vi "Obsever Structure.vi"(8 "error in (no error)":errorcluster, 11 "Vessel in":refnum<class "Vessel.lvclass">) -> (0 "error out":errorcluster, 3 "Vessel out":refnum<class "Vessel.lvclass">)   [LabVIEW 2014, in "Vessel.lvclass"]
doc: "This is the main running method that runs the control loop."
uses:
  Vessel.lvclass
  Observer/Observer.lvclass
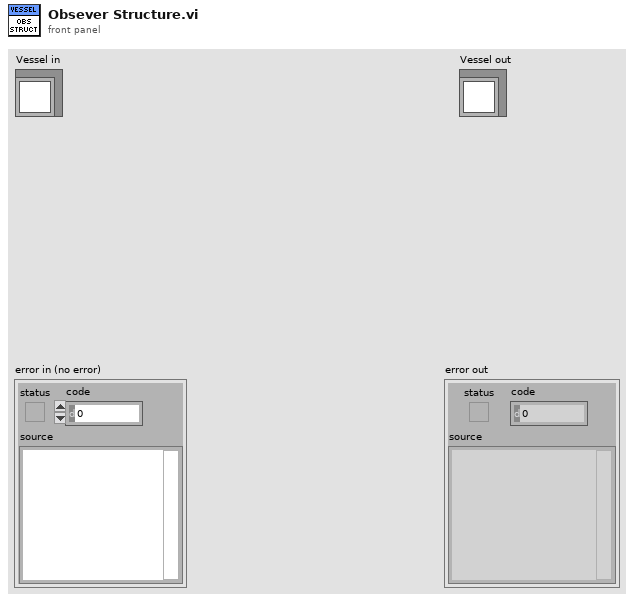
[diagram p1: front panel]
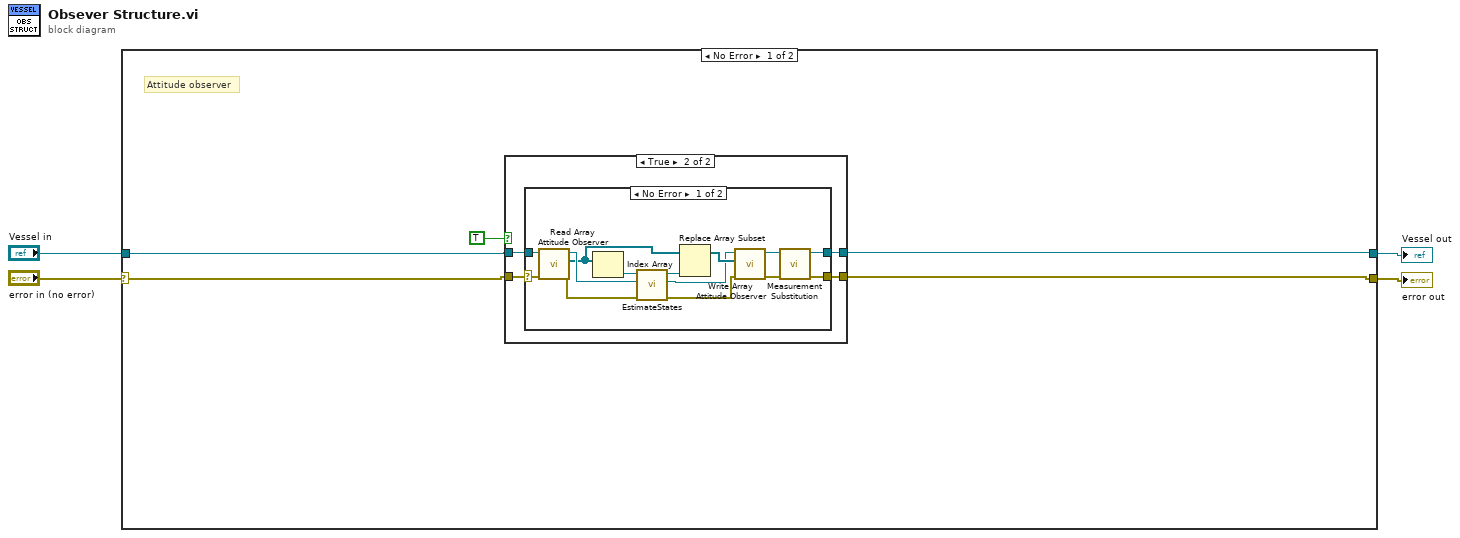
[diagram p0: block diagram]
diagram:
  n1 = case shown="No Error" "error in (no error)" {
    selector: "error in (no error)" -> [w8 w33]
    tunnel: [w6 w33] -> w3
    tunnel: [w7 w32] -> w1
    tunnel: "Vessel in" -> [w9 w32]
    frame No Error {
      # "Attitude observer"
      n2 = case shown="True" TRUE {
        tunnel: [w11 w15] -> w7
        tunnel: [w10 w14] -> w6
        tunnel: w9 -> [w11 w13]
        tunnel: w8 -> [w10 w12]
        frame False {
        }
        frame True {
          n3 = case shown="No Error" w12 {
            selector: w12 -> [w28 w30]
            tunnel: w13 -> [w29 w31]
            tunnel: [w20 w31] -> w15
            tunnel: [w16 w30] -> w14
            frame No Error {
              n4 = call-dynamic "Read Array Attitude Observer.vi"("error in (no error)"=w28, "Vessel in"=w29) -> ("error out"=w19:errorcluster, "Array Attitude Observer"=w24:refnum<class "Observer.lvclass">[], "Vessel out"=w26:refnum<class "Vessel.lvclass">)  [unwired: 7 in]
              n5 = Index Array(array=w24) -> (element=w27:refnum<class "Observer.lvclass">)  [unwired: 1 in]
              n6 = call-dynamic "EstimateStates.vi"("error in (no error)"=w19, "Vessel In"=w26, "Observer in"=w27) -> ("error out"=w18:errorcluster, "Vessel Out"=w22:refnum<class "Vessel.lvclass">, "Observer out"=w25:refnum<class "Observer.lvclass">)  [unwired: 6 in]
              n7 = Replace Array Subset(array=w24, new element=w25) -> (w23:refnum<class "Observer.lvclass">[])  [unwired: 1 in]
              n8 = call-dynamic "Write Array Attitude Observer.vi"("error in (no error)"=w18, "Array Attitude Observer"=w23, "Vessel in"=w22) -> ("error out"=w17:errorcluster, "Vessel out"=w21:refnum<class "Vessel.lvclass">)  [unwired: 7 in]
              n9 = call-dynamic "Measurement Substitution.vi"("error in (no error)"=w17, "Vessel in"=w21) -> ("error out"=w16:errorcluster, "Vessel out"=w20:refnum<class "Vessel.lvclass">)  [unwired: 8 in]
            }
            frame Error {
            }
          }
        }
      }
    }
    frame Error {
    }
  }
  "error out" <- w3
  "Vessel out" <- w1
